vi "Converpourcent2.vi"(11 "input variable":i16) -> (3 "output variable":u8)   [LabVIEW 2015]
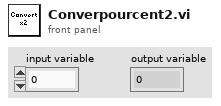
[diagram p1: front panel]
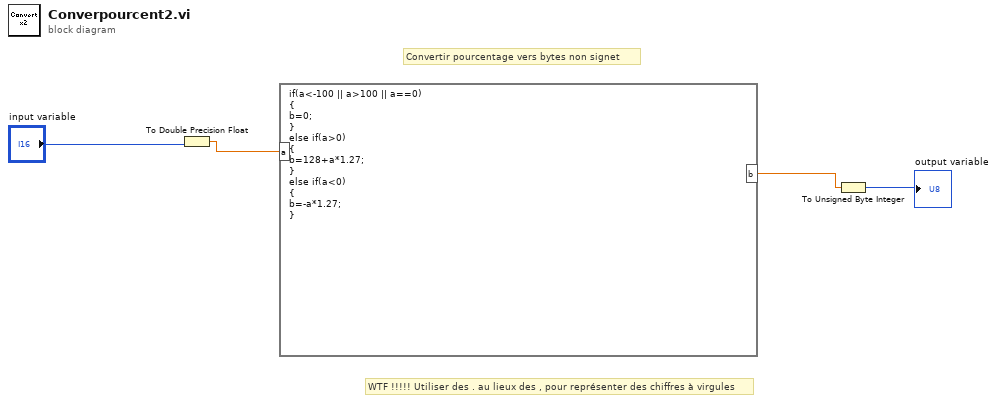
[diagram p0: block diagram]
diagram:
  # "WTF !!!!! Utiliser des . au lieux des , pour représenter des chiffres à virgules"
  # "Range value"
  # "Convertir pourcentage vers bytes non signet"
  n1 = To Double Precision Float(number="input variable") -> (double precision float=w1:dbl)
  n2 = formula code="if(a<-100 || a>100 || a==0)\n{\nb=0;\n}\nelse if(a>0)\n{\nb=128+a*1.27;\n}\nelse if(a<0)\n{\nb=-a*1.27;\n}"("a"=w1) -> ("b"=w3:dbl)
  n3 = To Unsigned Byte Integer(number=w3) -> (unsigned 8bit integer=→"output variable":u8)
